vi "Main.vi"(8 "error in (no error)":errorcluster, 11 "ChatBase in":refnum<class "Chat.lvclass">) -> (0 "error out":errorcluster, 3 "component":refnum<class "Chat.lvclass">)   [LabVIEW 2012, in "Chat.lvclass"]
doc: "Main VI of the component."
uses:
  Chat.lvclass
  person_cluster.ctl
  Chat.lvclass/Chat.ctl
  <vilib>/Distrio/Murmex/InitialiseMessage/InitialiseMessage.lvclass
  <vilib>/Distrio/Murmex/TerminateMessage/TerminateMessage.lvclass
  <vilib>/Distrio/Murmex/ConfigureMessage/ConfigureMessage.lvclass
  <vilib>/Distrio/Murmex/GenericMessage/GenericMessage.lvclass
  <vilib>/Distrio/Murmex/Murmex/Set configure at initialise.vi
  <vilib>/Distrio/Murmex/Murmex/Set VI reference.vi
  <vilib>/Distrio/Murmex/Murmex/Set log reference.vi
  <vilib>/Distrio/Murmex/Message/Add or replace parameter.vi
  <vilib>/Distrio/Murmex/Murmex/Murmex.lvclass
panel:
  in  "button:send":bool
  in  "people":T1[](array[typedef])
  out "message list":string
  in  "button:configure":bool
  in  "text:message":string
  in  "button:quit":bool
  out "terminate?":bool
  out "log":string
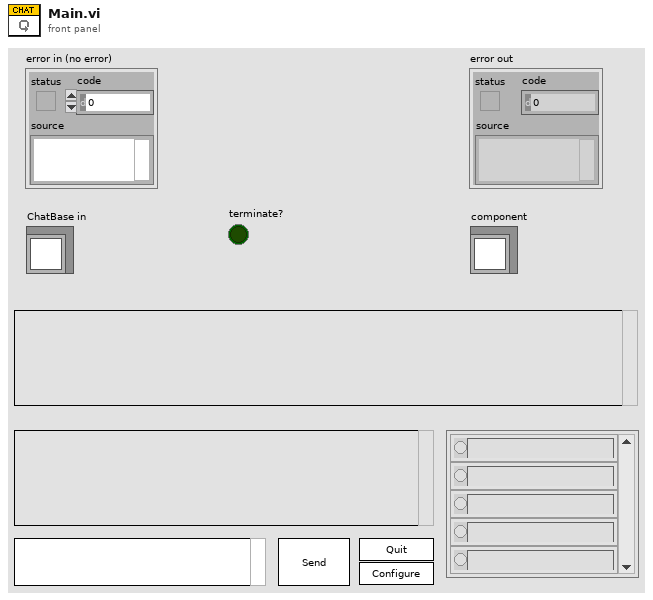
[diagram p1: front panel]
types:
  T1 = typedef "Chat.lvclass/person_cluster.ctl" = cluster{"writing?":bool, "name":string}
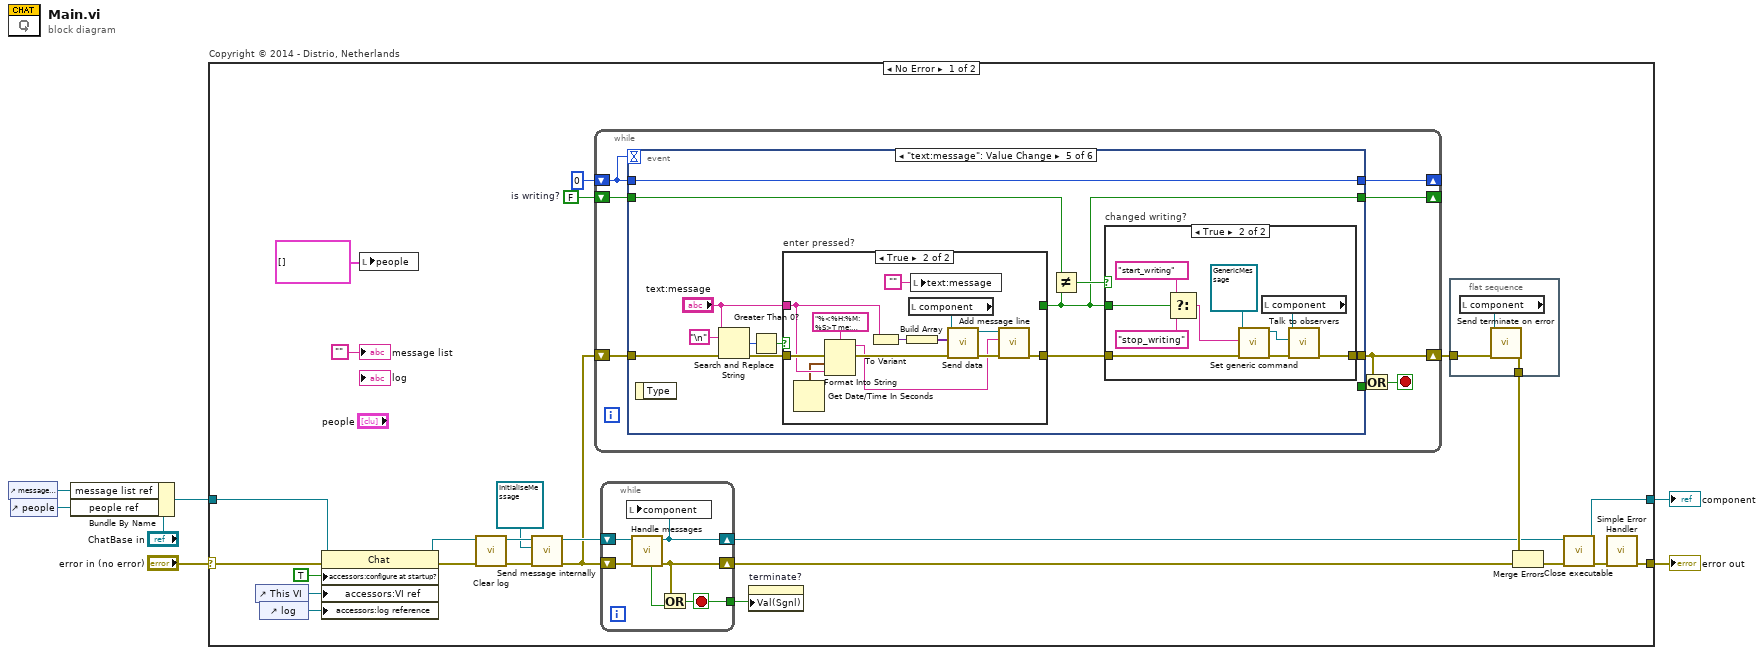
[diagram p0: block diagram]
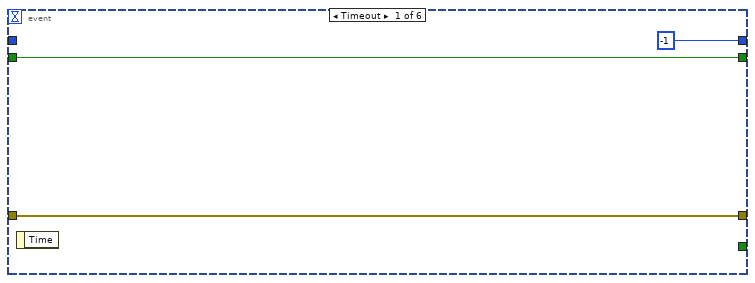
[diagram p2: hidden frame]
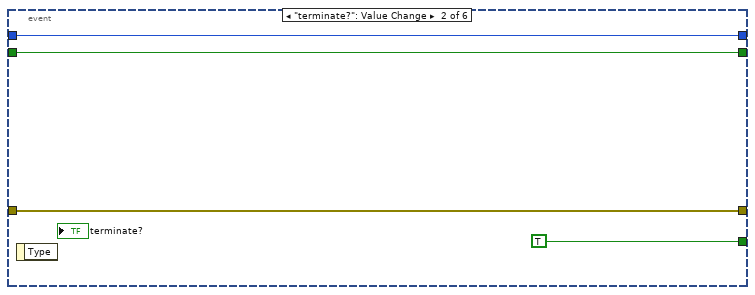
[diagram p3: hidden frame]
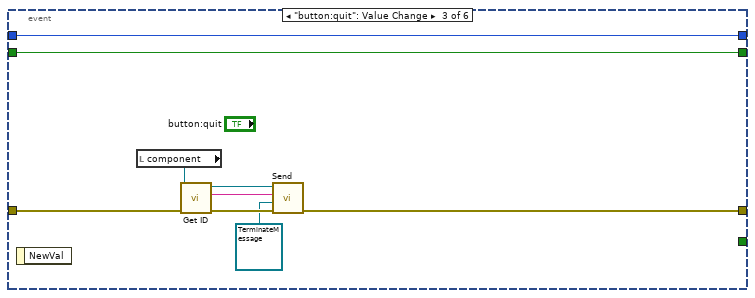
[diagram p4: hidden frame]
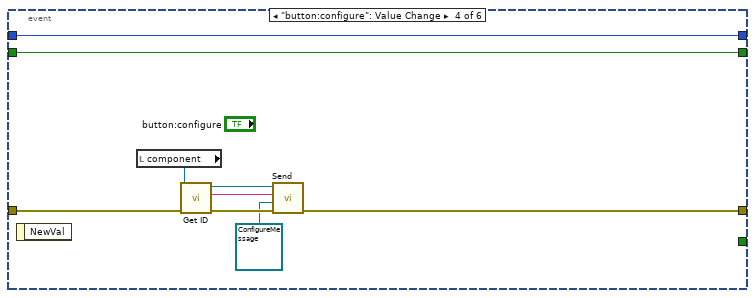
[diagram p5: hidden frame]
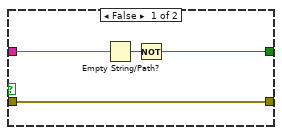
[diagram p7: hidden frame]
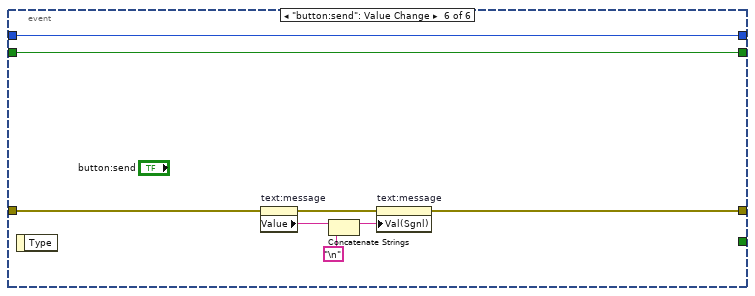
[diagram p8: hidden frame]
diagram:
  n1 = control-ref of="message list"() -> (w5:refnum<vi>)
  n2 = control-ref of="people"() -> (w2:refnum<vi>)
  n3 = Bundle By Name(cluster="ChatBase in", "message list ref"=w5, "people ref"=w2) -> (w3:refnum<class "Chat.lvclass">)
  n4 = case "Copyright © 2014 - Distrio, Netherlands" shown="No Error" "error in (no error)" {
    selector: "error in (no error)" -> [w12 w124]
    tunnel: [w9 w123] -> w7
    tunnel: [w32 w124] -> w6
    tunnel: w3 -> [w19 w123]
    frame No Error {
      w20 = FALSE  # is writing?
      n5 = control-ref of="This VI"() -> (w28:refnum<vi>)
      n6 = control-ref of="log"() -> (w27:refnum<vi>)
      n7 = property class="Chat"(reference=w19, error in=w12, "accessors:configure at startup?"=TRUE ("configure at startup?"), "accessors:VI ref"=w28, "accessors:log reference"=w27) -> (reference out=w22:refnum<class "Chat.lvclass">, error out=w31:errorcluster)
      n8 = local write "people"(T1[] [] ("people")) -> ()
      n9 = call <vilib>:"Clear log.vi"("error in (no error)"=w31, "MurmexBase in"=w22) -> ("error out"=w23:errorcluster, "MurmexBase out"=w21:refnum<class "Chat.lvclass">)  [unwired: 8 in]
      n10 = call <vilib>:"Send message internally.vi"("error in (no error)"=w23, "Message"=refnum<class "InitialiseMessage.lvclass"> refnum ("InitialiseMessage"), "Murmex in"=w21) -> ("error out"=w26:errorcluster, "Murmex out"=w30:refnum<class "Chat.lvclass">)  [unwired: 7 in]
      n11 = while {
        shift-right: [w42] -> _
        shift-left: 0 -> [w41]
        shift-right: [w40] -> w16
        shift-left: w26 -> [w43]
        shift-right: [w36] -> _
        shift-left: w20 -> [w37]
        stop <- w38 stop-if-true
        n12 = event shown="[4] \"text:message\": Value Change" {
          selector: _ -> [_ _ _ _ _ _]
          dyn-events: _ -> [_ _ _ _ _ _]
          timeout: w41 -> [_ _ _ _ _ _]
          tunnel: w43 -> [w46 w50 w58 w67 w77 w111]
          tunnel: [-1 w48 w59 w68 w80 w116] -> w42
          tunnel: w41 -> [_ w48 w59 w68 w80 w116]
          tunnel: [w46 w50 w57 w66 w71 w109] -> w40
          tunnel: [_ TRUE _ _ _ _] -> w39
          tunnel: w37 -> [w44 w47 w51 w61 w73 w115]
          tunnel: [w44 w47 w51 w61 w69 w115] -> w36
          event Timeout {
            n13 = event-data() -> ()  [unwired: 1 in, 1 out]
          }
          event "terminate?": Value Change {
            n14 = event-data() -> ()  [unwired: 1 in, 1 out]
          }
          event "button:quit": Value Change {
            n15 = event-data() -> ()  [unwired: 1 in, 1 out]
            n16 = local read "component"() -> (w54:refnum<class "Chat.lvclass">)
            n17 = call <vilib>:"Get ID.vi"("error in (no error)"=w58, "Murmex in"=w54) -> ("error out"=w56:errorcluster, "component id"=w53:string, "Murmex out"=w55:refnum<class "Chat.lvclass">)  [unwired: 7 in]
            n18 = call <vilib>:"Send.vi"("error in (no error)"=w56, "Message"=refnum<class "TerminateMessage.lvclass"> refnum ("TerminateMessage"), "recipient"=w53, "Murmex in"=w55) -> ("error out"=w57:errorcluster)  [unwired: 6 in, 1 out]
          }
          event "button:configure": Value Change {
            n19 = event-data() -> ()  [unwired: 1 in, 1 out]
            n20 = local read "component"() -> (w63:refnum<class "Chat.lvclass">)
            n21 = call <vilib>:"Get ID.vi"("error in (no error)"=w67, "Murmex in"=w63) -> ("error out"=w65:errorcluster, "component id"=w62:string, "Murmex out"=w64:refnum<class "Chat.lvclass">)  [unwired: 7 in]
            n22 = call <vilib>:"Send.vi"("error in (no error)"=w65, "Message"=refnum<class "ConfigureMessage.lvclass"> refnum ("ConfigureMessage"), "recipient"=w62, "Murmex in"=w64) -> ("error out"=w66:errorcluster)  [unwired: 6 in, 1 out]
          }
          event "text:message": Value Change {
            n23 = event-data() -> ()  [unwired: 1 in, 1 out]
            n24 = Search and Replace String(input string="text:message", search string="\n", error in=w77) -> (number of replacements=w79:i32, error out=w76:errorcluster)  [unwired: 5 in, 2 out]
            n25 = Greater Than 0?(x=w79) -> (x > 0?=w74:bool)
            n26 = case "enter pressed?" shown="True" w74 {
              tunnel: [w95 w102] -> w72
              tunnel: w76 -> [w95 w101]
              tunnel: "text:message" -> [w93 w99]
              tunnel: [w92 _] -> w69
              frame False {
                n27 = Empty String/Path?(string/path=w93) -> (empty?=w94:bool)
                n28 = Not(x=w94) -> (.not. x?=w92:bool)
              }
              frame True {
                n29 = Get Date/Time In Seconds() -> (seconds since 1Jan1904=w98:timestamp)
                n30 = Format Into String(format string="%<%H:%M:%S>T me: %s", error in=w101, w98, w99) -> (resulting string=w97:string, error out=w100:errorcluster)  [unwired: 1 in]
                n31 = To Variant(anything=w99) -> (Variant=w107:variant)
                n32 = Build Array(w107) -> (w106:variant[])
                n33 = local read "component"() -> (w108:refnum<class "Chat.lvclass">)
                n34 = local write "text:message"("") -> ()
                n35 = call <vilib>:"Send data.vi"("error in (no error)"=w100, "data (channels array)"=w106, "Murmex in"=w108) -> ("error out"=w103:errorcluster, "Murmex out"=w104:refnum<class "Chat.lvclass">)  [unwired: 7 in]
                n36 = call "Add message line.vi"("error in (no error)"=w103, "Message in"=w97, "Chat in"=w104) -> ("error out"=w102:errorcluster)  [unwired: 7 in, 1 out]
              }
            }
            n37 = Not Equal?(x=w73, y=w69) -> (x != y?=w70:bool)
            n38 = case "changed writing?" shown="True" w70 {
              tunnel: w72 -> [w81 w89]
              tunnel: [w81 w91] -> w71
              tunnel: w69 -> [_ w85]
              frame False {
              }
              frame True {
                n39 = Select(t="start_writing" ("generic command"), s=w85, f="stop_writing" ("generic command")) -> (s? t:f=w83:string)
                n40 = call <vilib>:"Set generic command.vi"("error in (no error)"=w89, "generic command"=w83, "GenericMessage in"=refnum<class "GenericMessage.lvclass"> refnum ("GenericMessage")) -> ("error out"=w88:errorcluster, "GenericMessage out"=w86:refnum<class "GenericMessage.lvclass">)  [unwired: 7 in]
                n41 = local read "component"() -> (w90:refnum<class "Chat.lvclass">)
                n42 = call <vilib>:"Talk to observers.vi"("error in (no error)"=w88, "Message"=w86, "Murmex in"=w90) -> ("error out"=w91:errorcluster)  [unwired: 7 in, 1 out]
              }
            }
          }
          event "button:send": Value Change {
            n43 = event-data() -> ()  [unwired: 1 in, 1 out]
            n44 = property on="text:message" class="Str"(error in=w111) -> (error out=w110:errorcluster, "Value"=w114:string)  [unwired: 1 in, 1 out]
            n45 = Concatenate Strings(w114, "\n") -> (w112:string)
            n46 = property on="text:message" class="Str"(error in=w110, "Val(Sgnl)"=w112) -> (error out=w109:errorcluster)  [unwired: 1 in, 1 out]
          }
        }
        n47 = Or(x=w40, y=w39) -> (x .or. y?=w38:bool)
      }
      n48 = while {
        shift-right: [w118] -> w14
        shift-left: w26 -> [w122]
        shift-right: [w117] -> w10
        shift-left: w30 -> [w121]
        tunnel: [w119] -> w24
        stop <- w119 stop-if-true
        n49 = call <vilib>:"Handle messages.vi"("error in (no error)"=w122, "Murmex in"=w121) -> ("error out"=w118:errorcluster, "Murmex out"=w117:refnum<class "Chat.lvclass">, "terminated?"=w120:bool)  [unwired: 7 in]
        n50 = local write "component"(w117) -> ()
        n51 = Or(x=w118, y=w120) -> (x .or. y?=w119:bool)
      }
      n52 = property on="terminate?" class="Bool (strict)"("Val(Sgnl)"=w24) -> ()  [unwired: 2 in, 2 out]
      n53 = flat-sequence {
        tunnel: w16 -> [w35]
        tunnel: [w34] -> w15
        frame #0 {
          n54 = local read "component"() -> (w33:refnum<class "Chat.lvclass">)
          n55 = call <vilib>:"Send terminate on error.vi"("error in (no error)"=w35, "Murmex in"=w33) -> ("error out"=w34:errorcluster)  [unwired: 8 in, 1 out]
        }
      }
      n56 = Merge Errors(w15, w14) -> (w13:errorcluster)
      n57 = call <vilib>:"Close executable.vi"("error in (no error)"=w13, "MurmexBase in"=w10) -> ("error out"=w11:errorcluster, "MurmexBase out"=w9:refnum<class "Chat.lvclass">)  [unwired: 8 in]
      n58 = call <vilib>:"Simple Error Handler.vi"("error in (no error)"=w11) -> ("error out"=w32:errorcluster)  [unwired: 4 in, 4 out]
      "message list" <- ""
    }
    frame Error {
    }
  }
  "error out" <- w6
  "component" <- w7
